vi "GetResultScaleAndOffset.vi"(11 "MeasureConfig":T1={"Bead locations"=[{"X"=0, "Y"=0}], "ROI"=200, "Experiment base path"=path "", "Image output subdir"="images", "Output mode"=enum."None", "Traces output subdir"="traces", "QTrk Settings"={"Image width"=150, "Image height"=150, "Number of threads (CPU based)"=-1, "CUDA Device"=-2, "COM Background correction factor"=0.0, "ZLUT MinRadius"=8.0, "ZLUT Radial sample density"=5.0, "ZLUT Angular sample density"=2.0, "ZLUT ROI Coverage"=0.7, "QI Iterations"=1, "QI MinRadius"=2.0, "QI Radial sample density"=5.0, "QI Angular sample density"=2.0, "QI ROI Coverage"=0.7, "QI Angular Step \nIteration Factor"=0.8, "XCOR Profile Length"=1, "XCOR Profile Width"=128, "XCOR Iterations"=32, "Gaussian 2D Fit Iterations"=2, "Gaussian 2D Sigma (pixels)"=3.0}, "Tracking Config"={"Number of steps"=0, "ZLUT stepsize (um)"=0.0, "Z correction factor"=0.0, "Start piezo Z (um)"=0.0, "Pixel size (nm)"=0.0, "2D Localization Type"=enum."Quadrant Interpolation", "Z Command (None)"=enum."ComputeZ", "Z Piezo scale"=FALSE}, "Experiment Name"="", "Program"={"Commands"=[], "Motor Axis accuracy conditions"={"Magnet Z"=0.0, "Magnet rotation"=0.0, "Camera"={"X"=0.0, "Y"=0.0}, "Piezo XY"={"X"=0.0, "Y"=0.0}, "Piezo Z"=0.0}, "Axis flags"={"Magnet Z"=FALSE, "Magnet rotation"=FALSE, "Camera"={"X"=FALSE, "Y"=FALSE}, "Piezo XY"={"X"=FALSE, "Y"=FALSE}, "Piezo Z"=FALSE}}, "ZLUT"=[], "Camera settings"={"Framerate (Hz)"=60, "Exposure time (us)"=5000, "Image size"={"Width"=1280, "Height"=1024}, "Number of buffers"=30}, "Experiment Script"="", "Max frames in memory"=2, "Save traces as binary"=FALSE, "Pixel Calibration Gain Image"="camera_calib_gain.bin", "Pixel Calibration Offset Image"="camera_calib_gain.bin", "Use pixel calibration images"=FALSE, "Internal camera settings"=""} {"QTrk Settings"."QI ROI Coverage" format="%_2g"; "QTrk Settings"."QI MinRadius" format="%.2f"; "QTrk Settings"."QI Angular sample density" format="%.3f"; "QTrk Settings"."QI Radial sample density" format="%.2f"; "QTrk Settings"."ZLUT Radial sample density" format="%.2f"; "QTrk Settings"."ZLUT MinRadius" format="%.2f"}) -> (2 "offset":cluster{dbl, dbl, "y":sgl}, 3 "scale":cluster{sgl, sgl, sgl})   [LabVIEW 2011]
uses:
  Typedefs/MeasureConfigType.ctl
  Typedefs/MeasureConfigOutputMode.ctl
  qtrk/QTrk.llb/QTrkSettings.ctl
  Typedefs/TrackingConfigType.ctl
  qtrk/QTrk.llb/QTrkLocalizationType.ctl
  qtrk/QTrk.llb/QTrkZCommandType.ctl
  ExperimentProgram/ExperimentProgramType.ctl
  ExperimentProgram/ExProgCommandType.ctl
  ExperimentProgram/ExProgCommandEnumType.ctl
  Motors/MotorAxisEnum.ctl
  Motors/MotorPosType.ctl
  Typedefs/XYf.ctl
  Motors/MotorPosFlagsType.ctl
  Camera/GenericCameraConfigType.ctl
panel:
  # "(used for commands with string parameters)"
  # "-2: Use all devices\n-1: Use best device"
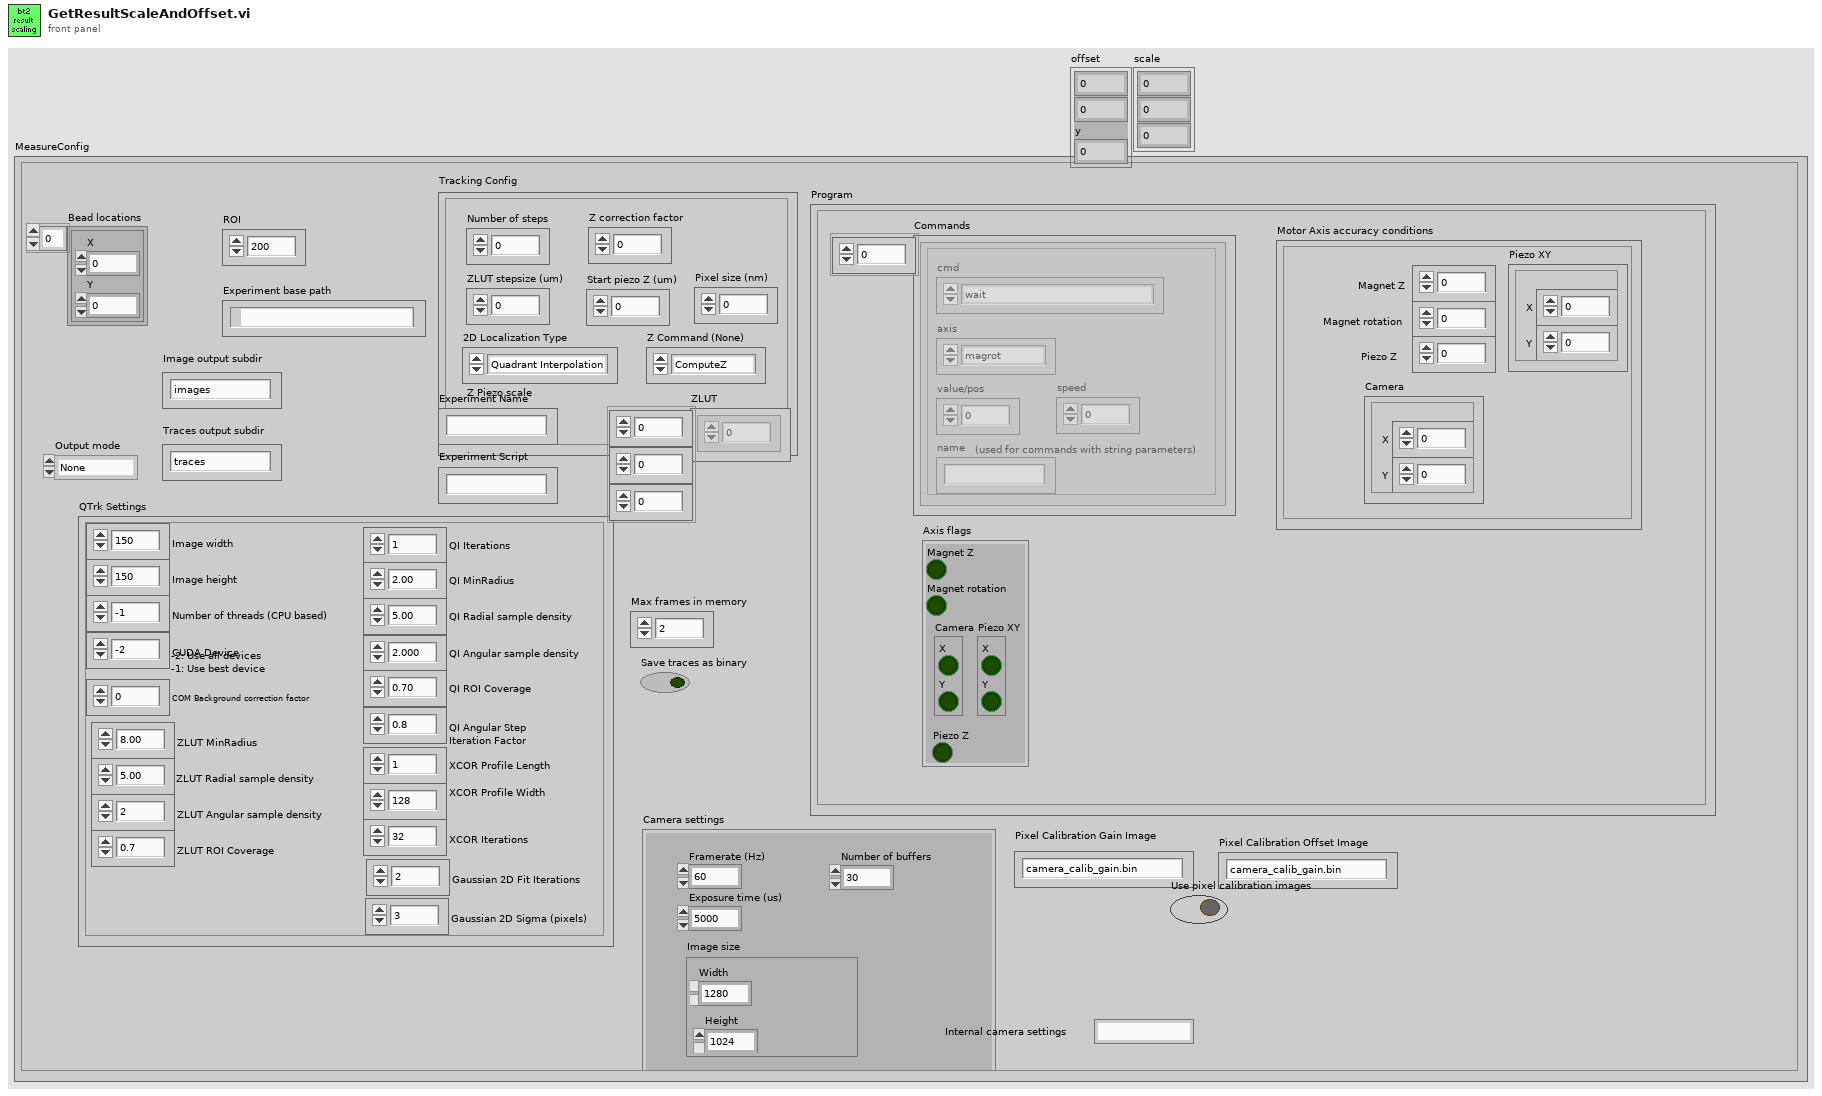
[diagram p1: front panel]
types:
  T1 = typedef "MeasureConfigType.ctl" = cluster{"Bead locations":cluster{"X":i32, "Y":i32}[], "ROI":i32, "Experiment base path":path, "Image output subdir":string, "Output mode":T2, "Traces output subdir":string, "QTrk Settings":T3, "Tracking Config":T4, "Experiment Name":string, "Program":T7, "ZLUT":sgl[][][], "Camera settings":T14, "Experiment Script":string, "Max frames in memory":i32, "Save traces as binary":bool, "Pixel Calibration Gain Image":string, "Pixel Calibration Offset Image":string, "Use pixel calibration images":bool, "Internal camera settings":string}
  T2 = typedef "MeasureConfigOutputMode.ctl" = enum16{"None", "Track", "SaveImages"}
  T3 = typedef "QTrkSettings.ctl" = cluster{"Image width":i32, "Image height":i32, "Number of threads (CPU based)":i32, "CUDA Device":i32, "COM Background correction factor":sgl, "ZLUT MinRadius":sgl, "ZLUT Radial sample density":sgl, "ZLUT Angular sample density":sgl, "ZLUT ROI Coverage":sgl, "QI Iterations":i32, "QI MinRadius":sgl, "QI Radial sample density":sgl, "QI Angular sample density":sgl, "QI ROI Coverage":sgl, "QI Angular Step \nIteration Factor":sgl, "XCOR Profile Length":i32, "XCOR Profile Width":i32, "XCOR Iterations":i32, "Gaussian 2D Fit Iterations":i32, "Gaussian 2D Sigma (pixels)":sgl}
  T4 = typedef "TrackingConfigType.ctl" = cluster{"Number of steps":i32, "ZLUT stepsize (um)":sgl, "Z correction factor":sgl, "Start piezo Z (um)":sgl, "Pixel size (nm)":sgl, "2D Localization Type":T5, "Z Command (None)":T6, "Z Piezo scale":bool}
  T5 = typedef "QTrkLocalizationType.ctl" = enum16{"Center-of-Mass", "1D Cross-Correlation", "Quadrant Interpolation", "Gaussian 2D MLE", "QI + ZLUTAlign", "ZLUTAlign"}
  T6 = typedef "QTrkZCommandType.ctl" = enum16{"Nothing", "ComputeZ", "BuildRadialZLUT", "BuildImageZLUT", "RadialZLUT+ImageZLUT"}
  T7 = typedef "ExperimentProgramType.ctl" = cluster{"Commands":T8[], "Motor Axis accuracy conditions":T11, "Axis flags":T13}
  T8 = typedef "ExProgCommandType.ctl" = cluster{"cmd":T9, "axis":T10, "value/pos":dbl, "speed":dbl, "name":string}
  T9 = typedef "ExProgCommandEnumType.ctl" = enum16{"wait", "move", "acquire", "idle", "rmove", "when", "section", "stop"}
  T10 = typedef "MotorAxisEnum.ctl" = enum16{"no axis", "magrot", "magpos", "px", "py", "pz", "camx", "camy"}
  T11 = typedef "MotorPosType.ctl" = cluster{"Magnet Z":dbl, "Magnet rotation":dbl, "Camera":T12, "Piezo XY":T12, "Piezo Z":dbl}
  T12 = typedef "XYf.ctl" = cluster{"X":sgl, "Y":sgl}
  T13 = typedef "MotorPosFlagsType.ctl" = cluster{"Magnet Z":bool, "Magnet rotation":bool, "Camera":cluster{"X":bool, "Y":bool}, "Piezo XY":cluster{"X":bool, "Y":bool}, "Piezo Z":bool}
  T14 = typedef "GenericCameraConfigType.ctl" = cluster{"Framerate (Hz)":i32, "Exposure time (us)":i32, "Image size":cluster{"Width":i32, "Height":i32}, "Number of buffers":i32}
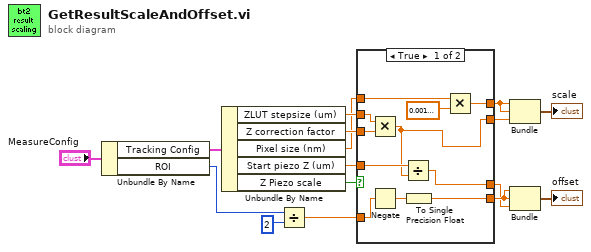
[diagram p0: block diagram]
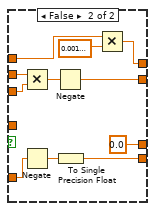
[diagram p2: hidden frame]
diagram:
  n1 = Unbundle By Name("MeasureConfig") -> ("Tracking Config"=w15:T4, "ROI"=w14:i32)
  n2 = Unbundle By Name(w15) -> ("ZLUT stepsize (um)"=w12:sgl, "Z correction factor"=w11:sgl, "Pixel size (nm)"=w10:sgl, "Start piezo Z (um)"=w4:sgl, "Z Piezo scale"=w1:bool)
  n3 = Divide(x=w14, y=2) -> (x/y=w8:dbl)
  n4 = case shown="True" w1 {
    tunnel: w12 -> [w27 w38]
    tunnel: w11 -> [w26 w37]
    tunnel: w10 -> [w25 w36]
    tunnel: [w23 w34] -> w9
    tunnel: w8 -> [w22 w33]
    tunnel: [w20 w31] -> w5
    tunnel: w4 -> [w19 _]
    tunnel: [w17 w29] -> w3
    tunnel: [w18 sgl 0.0] -> w2
    frame True {
      n5 = Multiply(x=w27, y=w26) -> (x*y=w17:sgl)
      n6 = Negate(x=w22) -> (-x=w21:dbl)
      n7 = Divide(x=w19, y=w17) -> (x/y=w18:sgl)
      n8 = To Single Precision Float(number=w21) -> (single precision float=w20:sgl)
      n9 = Multiply(x=w25, y=sgl 0.001) -> (x*y=w23:sgl)
    }
    frame False {
      n10 = Multiply(x=w38, y=w37) -> (x*y=w30:sgl)
      n11 = Negate(x=w33) -> (-x=w32:dbl)
      n12 = Negate(x=w30) -> (-x=w29:sgl)
      n13 = To Single Precision Float(number=w32) -> (single precision float=w31:sgl)
      n14 = Multiply(x=w36, y=sgl 0.001) -> (x*y=w34:sgl)
    }
  }
  n15 = Bundle(w9, w9, w3) -> (→"scale":cluster{sgl, sgl, sgl})  [unwired: 1 in]
  n16 = Bundle(w5, w5, w2) -> (→"offset":cluster{sgl, sgl, sgl})  [unwired: 1 in]
